vi "SetupArea.vi"(8 "error in (no error)":errorcluster) -> (0 "error out":errorcluster)   [LabVIEW 2015, in "ESLSCDLL.lvlib"]
uses:
  ESLSCDLL.lvlib
  Globals.vi
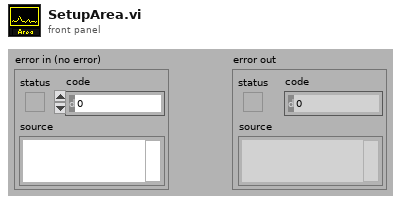
[diagram p1: front panel]
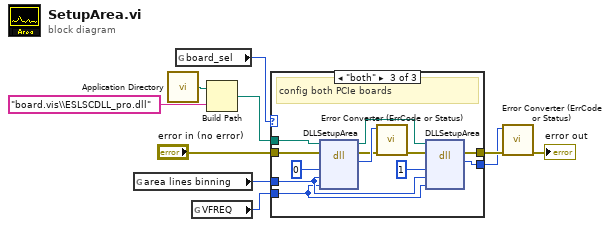
[diagram p0: block diagram]
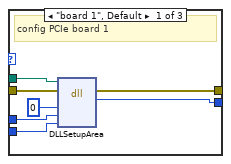
[diagram p2: hidden frame]
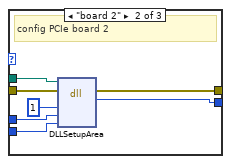
[diagram p3: hidden frame]
diagram:
  n1 = global read "Globals.vi" "area lines binning"() -> (w4:u32)
  n2 = call <vilib>:"Application Directory.vi"() -> ("Application Directory"=w3:path)
  n3 = global read "Globals.vi" "board_sel"() -> (w6:enum16{"0", "board 1", "board 2", "both"})
  n4 = global read "Globals.vi" "VFREQ"() -> (w5:u32)
  n5 = Build Path(base path=w3, name or relative path="board.vis\\ESLSCDLL_pro.dll") -> (appended path=w1:path)
  n6 = case shown="\"both\"" w6 {
    tunnel: w4 -> [w17 w24 w34]
    tunnel: w5 -> [w16 w23 w33]
    tunnel: "error in (no error)" -> [w15 w22 w30]
    tunnel: [w14 w21 w28] -> w8
    tunnel: [w13 w20 w27] -> w7
    tunnel: w1 -> [w12 w19 w26]
    frame "board 1", Default {
      # "config PCIe board 1"
      n7 = dll-call lib="C:/ENTW/PCIE/LV64/board.vis/ESLSCDLL_pro.dll" fn="DLLSetupArea" ("lwlscdll.dll:DLLReadFFLoop")(path in=w12, error in=w15, "drvno"=u32 0, "lines_binning"=w17, "vfreq"=w16) -> (error out=w14:errorcluster, "es_status_codes"=w13:i32)  [unwired: 4 in, 1 out]
    }
    frame "board 2" {
      # "config PCIe board 2"
      n8 = dll-call lib="C:/ENTW/PCIE/LV64/board.vis/ESLSCDLL_pro.dll" fn="DLLSetupArea" ("lwlscdll.dll:DLLReadFFLoop")(path in=w19, error in=w22, "drvno"=u32 1, "lines_binning"=w24, "vfreq"=w23) -> (error out=w21:errorcluster, "es_status_codes"=w20:i32)  [unwired: 4 in, 1 out]
    }
    frame "both" {
      # "config both PCIe boards"
      n9 = dll-call lib="C:/ENTW/PCIE/LV64/board.vis/ESLSCDLL_pro.dll" fn="DLLSetupArea" ("lwlscdll.dll:DLLReadFFLoop")(path in=w26, error in=w30, "drvno"=u32 0, "lines_binning"=w34, "vfreq"=w33) -> (path out=w25:path, error out=w31:errorcluster, "es_status_codes"=w32:i32)  [unwired: 4 in]
      n10 = call "Error Converter (ErrCode or Status).vi"("error in (no error)"=w31, "error code"=w32) -> ("error out"=w29:errorcluster)  [unwired: 9 in]
      n11 = dll-call lib="C:/ENTW/PCIE/LV64/board.vis/ESLSCDLL_pro.dll" fn="DLLSetupArea" ("lwlscdll.dll:DLLReadFFLoop")(path in=w25, error in=w29, "drvno"=u32 1, "lines_binning"=w34, "vfreq"=w33) -> (error out=w28:errorcluster, "es_status_codes"=w27:i32)  [unwired: 4 in, 1 out]
    }
  }
  n12 = call "Error Converter (ErrCode or Status).vi"("error in (no error)"=w8, "error code"=w7) -> ("error out"=→"error out":errorcluster)  [unwired: 9 in]
